vi "HOST.vi"(8 "Стоп":bool, 9 "Стоп GoTo":bool, 10 "Погнали!":bool, 11 "Куда едем?":T1(ring)) -> (3 "Текущая позиция":dbl)   [LabVIEW 2018]
uses:
  Spels.AutomationTools.Utility.Wcf.dll
  AmateurStepperMotor.dll
panel:
  out "Готово":bool
  in  "Тест":bool
  in  "Стоп_тест":bool
  in  "StepMultiplicationFactor":dbl=1.0
  in  "StepDivisor":i32(ring)=8 items=["D1"=1, "D2"=2, "D4"=4, "D8"=8, "D16"=16, "D32"=32]
  in  "Speed":dbl=1000.0
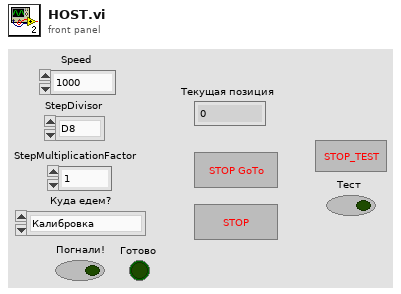
[diagram p1: front panel]
types:
  T1 = enum16{"Калибровка", "Первое стекло", "Второе стекло", "Третье стекло", "Четвертое стекло"}
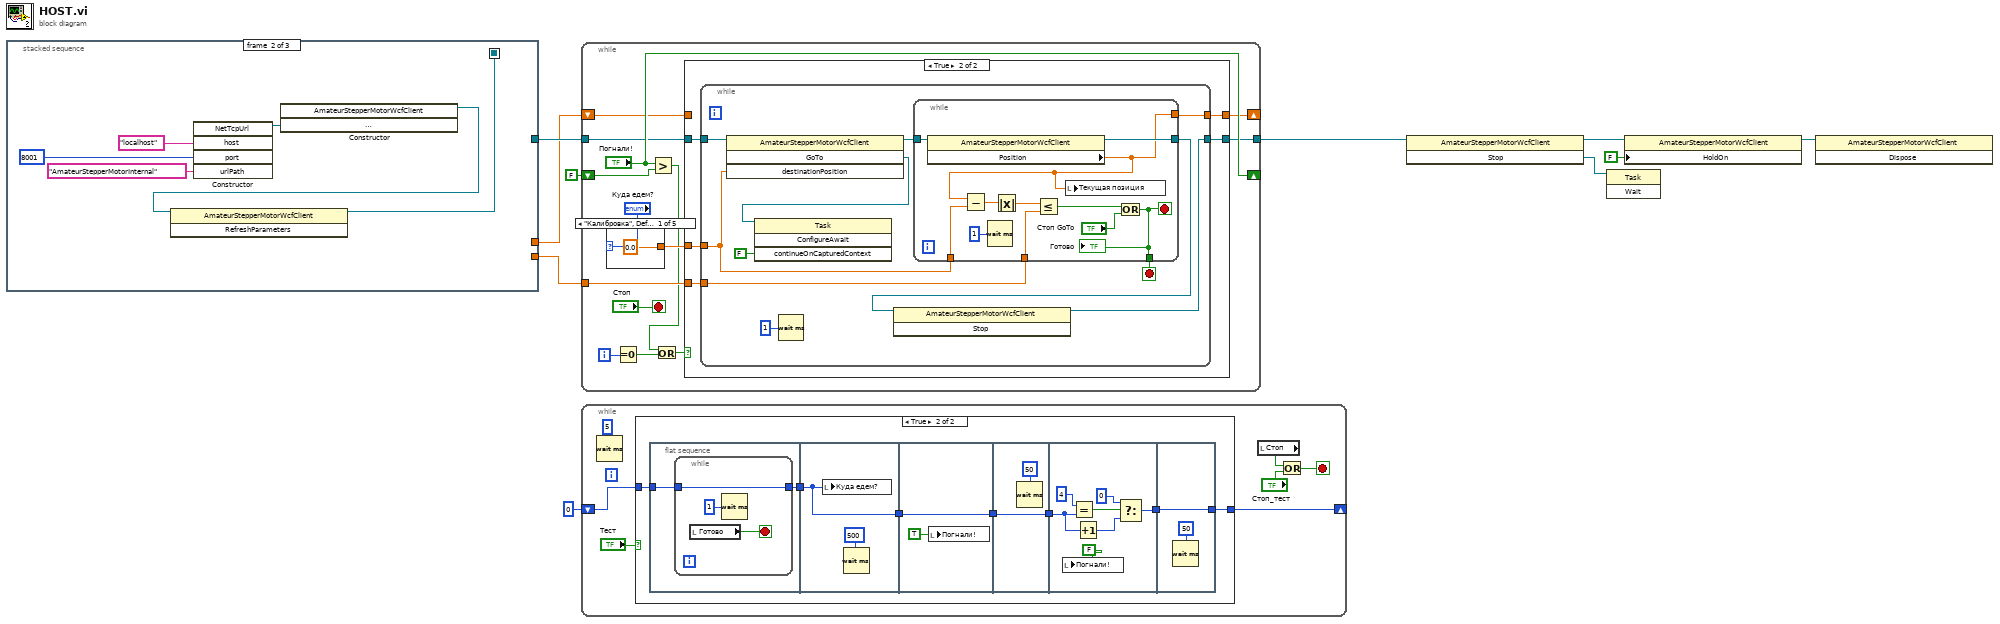
[diagram p0: block diagram]
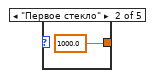
[diagram p3: hidden frame]
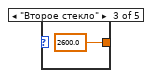
[diagram p4: hidden frame]
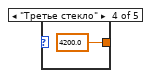
[diagram p5: hidden frame]
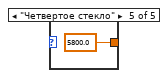
[diagram p6: hidden frame]
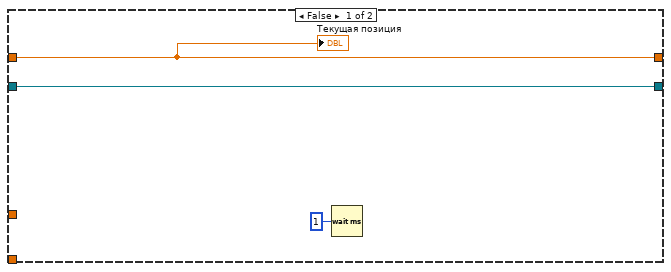
[diagram p7: hidden frame]
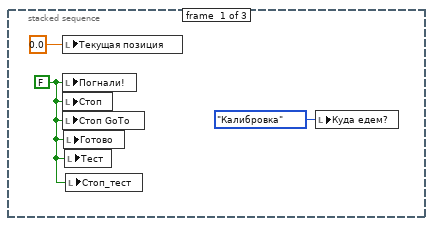
[diagram p8: hidden frame]
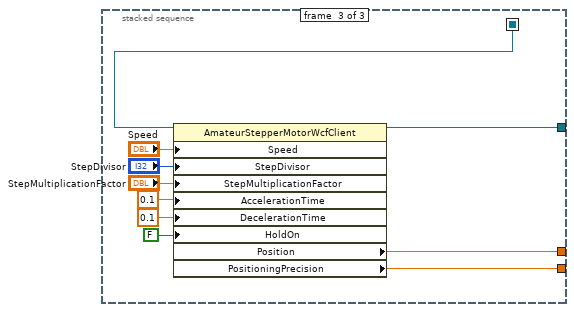
[diagram p9: hidden frame]
diagram:
  n1 = stacked-sequence {
    seq-local: [_ w14 _] -> [_ _ w26]
    tunnel: [_ _ w25] -> w6
    tunnel: [_ _ w21] -> w4
    tunnel: [_ _ w20] -> w3
    frame #0 {
      w12 = FALSE
      n2 = local write "Текущая позиция"(0.0 ("Текущая позиция")) -> ()
      n3 = local write "Погнали!"(w12) -> ()
      n4 = local write "Стоп"(w12) -> ()
      n5 = local write "Стоп GoTo"(w12) -> ()
      n6 = local write "Готово"(w12) -> ()
      n7 = local write "Тест"(w12) -> ()
      n8 = local write "Стоп_тест"(w12) -> ()
      n9 = local write "Куда едем?"(T1."Калибровка" ("Куда едем?")) -> ()
    }
    frame #1 {
      n10 = constructor class="NetTcpUrl"("host"="localhost", "port"=u32 8001, "urlPath"="AmateurStepperMotorInternal") -> (reference out=w16:refnum<k24>)  [unwired: 3 in, 5 out]
      n11 = constructor class="AmateurStepperMotorWcfClient"("serviceUrl"=w16) -> (reference out=w15:refnum<k24>)  [unwired: 3 in, 3 out]
      n12 = invoke class="AmateurStepperMotorWcfClient" method="RefreshParameters"(reference=w15) -> (reference out=w14:refnum<k24>)  [unwired: 2 in, 2 out]
    }
    frame #2 {
      n13 = property class="AmateurStepperMotorWcfClient"(reference=w26, "Speed"="Speed", "StepDivisor"="StepDivisor", "StepMultiplicationFactor"="StepMultiplicationFactor", "AccelerationTime"=0.1, "DecelerationTime"=0.1, "HoldOn"=FALSE) -> (reference out=w25:refnum<k24>, "Position"=w21:dbl, "PositioningPrecision"=w20:dbl)  [unwired: 1 in, 1 out]
    }
  }
  n14 = while {
    tunnel: w6 -> [w40]
    shift-right: ["Погнали!"] -> _
    shift-left: FALSE ("Поехали!") -> [w42]
    tunnel: [w39] -> w5
    shift-right: [w37] -> _
    shift-left: w4 -> [w38]
    tunnel: w3 -> [w36]
    i -> [w32]
    stop <- "Стоп" stop-if-true
    n15 = case shown="\"Калибровка\", Default" "Куда едем?" {
      tunnel: [0.0 1000.0 2600.0 4200.0 5800.0] -> w34
      frame "Калибровка", Default {
      }
      frame "Первое стекло" {
      }
      frame "Второе стекло" {
      }
      frame "Третье стекло" {
      }
      frame "Четвертое стекло" {
      }
    }
    n16 = Equal To 0?(x=w32) -> (x = 0?=w31:bool)
    n17 = Greater?(x="Погнали!", y=w42) -> (0:w30:bool)
    n18 = Or(x=w30, y=w31) -> (x .or. y?=w33:bool)
    n19 = case shown="True" w33 {
      tunnel: w34 -> [_ w56]
      tunnel: w40 -> [w50 w55]
      tunnel: [w50 w54] -> w39
      tunnel: w38 -> [w49 _]
      tunnel: [w49 w53] -> w37
      tunnel: w36 -> [_ w52]
      frame False {
        n20 = Wait (ms)(milliseconds to wait=u32 1) -> ()  [unwired: 1 out]
        "Текущая позиция" <- w49
      }
      frame True {
        n21 = while {
          tunnel: w56 -> [w61]
          tunnel: w55 -> [w64]
          tunnel: [w58] -> w54
          tunnel: [w63] -> w53
          tunnel: w52 -> [w60]
          stop <- w62 stop-if-true
          n22 = invoke class="AmateurStepperMotorWcfClient" method="GoTo"(reference=w64, "destinationPosition"=w61) -> (reference out=w66:refnum<k24>, "GoTo"=w67:refnum<k24>)  [unwired: 2 in, 2 out]
          n23 = invoke class="Task" method="ConfigureAwait"(reference=w67, "continueOnCapturedContext"=FALSE) -> ()  [unwired: 2 in, 4 out]
          n24 = Wait (ms)(milliseconds to wait=u32 1) -> ()  [unwired: 1 out]
          n25 = while {
            tunnel: [w70] -> w63
            tunnel: w66 -> [w78]
            tunnel: [w77] -> w59
            tunnel: [w69] -> w62
            tunnel: w61 -> [w75]
            tunnel: w60 -> [w73]
            stop <- w69 stop-if-true
            n26 = property class="AmateurStepperMotorWcfClient"(reference=w78) -> (reference out=w77:refnum<k24>, "Position"=w70:dbl)  [unwired: 1 in, 1 out]
            n27 = Subtract(x=w70, y=w75) -> (x-y=w76:dbl)
            n28 = Wait (ms)(milliseconds to wait=u32 1) -> ()  [unwired: 1 out]
            n29 = Absolute Value(x=w76) -> (abs(x)=w74:dbl)
            n30 = Less Or Equal?(x=w74, y=w73) -> (x <= y?=w72:bool)
            n31 = local write "Текущая позиция"(w70) -> ()
            n32 = Or(x=w72, y="Стоп GoTo") -> (x .or. y?=w69:bool)
            "Готово" <- w69
          }
          n33 = invoke class="AmateurStepperMotorWcfClient" method="Stop"(reference=w59) -> (reference out=w58:refnum<k24>)  [unwired: 2 in, 2 out]
        }
      }
    }
  }
  n34 = while {
    shift-right: [w79] -> _
    shift-left: 0 -> [w80]
    stop <- w83 stop-if-true
    n35 = Wait (ms)(milliseconds to wait=u32 5) -> ()  [unwired: 1 out]
    n36 = case shown="True" "Тест" {
      tunnel: w80 -> [w86 w93]
      tunnel: [w86 w90] -> w79
      frame False {
      }
      frame True {
        n37 = flat-sequence {
          tunnel: w93 -> [w95]
          tunnel: [w94] -> w88
          tunnel: [w100] -> w89
          tunnel: w88 -> [w100]
          tunnel: [w102] -> w91
          tunnel: w89 -> [w102]
          tunnel: [w103] -> w92
          tunnel: w91 -> [w103]
          tunnel: w92 -> [w108]
          tunnel: [w106] -> w87
          tunnel: [w113] -> w90
          tunnel: w87 -> [w113]
          frame #0 {
            n38 = while {
              tunnel: w95 -> [w98]
              tunnel: [w98] -> w94
              stop <- w97 stop-if-true
              n39 = local read "Готово"() -> (w97:bool)
              n40 = Wait (ms)(milliseconds to wait=u32 1) -> ()  [unwired: 1 out]
            }
          }
          frame #1 {
            n41 = local write "Куда едем?"(w100) -> ()
            n42 = Wait (ms)(milliseconds to wait=u32 500) -> ()  [unwired: 1 out]
          }
          frame #2 {
            n43 = local write "Погнали!"(TRUE ("Погнали!")) -> ()
          }
          frame #3 {
            n44 = Wait (ms)(milliseconds to wait=u32 50) -> ()  [unwired: 1 out]
          }
          frame #4 {
            n45 = local write "Погнали!"(FALSE ("Погнали!")) -> ()
            n46 = Equal?(x=4, y=w108) -> (x = y?=w110:bool)
            n47 = Increment(x=w108) -> (x+1=w107:i32)
            n48 = Select(t=0, s=w110, f=w107) -> (s? t:f=w106:i32)
          }
          frame #5 {
            n49 = Wait (ms)(milliseconds to wait=u32 50) -> ()  [unwired: 1 out]
          }
        }
      }
    }
    n50 = local read "Стоп"() -> (w82:bool)
    n51 = Or(x=w82, y="Стоп_тест") -> (x .or. y?=w83:bool)
  }
  n52 = invoke class="AmateurStepperMotorWcfClient" method="Stop"(reference=w5) -> (reference out=w9:refnum<k24>, "Stop"=w10:refnum<k24>)  [unwired: 2 in, 1 out]
  n53 = invoke class="Task" method="Wait"(reference=w10) -> ()  [unwired: 2 in, 3 out]
  n54 = property class="AmateurStepperMotorWcfClient"(reference=w9, "HoldOn"=FALSE) -> (reference out=w8:refnum<k24>)  [unwired: 1 in, 1 out]
  n55 = invoke class="AmateurStepperMotorWcfClient" method="Dispose"(reference=w8) -> ()  [unwired: 2 in, 3 out]
